vi "GetDeviceReference.vi"(8 "error in (no error)":errorcluster, 10 "Timeout(10s)":i32=10) -> (0 "error out":errorcluster, 3 "MainDevice Reference":refnum<k24>)   [LabVIEW 2019, in "LabNation Scope Driver.lvlib"]
doc: "Acquires the main device reference from the device manager. The reference Identifies the scope for all further actions."
uses:
  LabNation Scope Driver.lvlib
  <vilib>/Utility/error.llb/Error Cluster From Error Code.vi
  <vilib>/ErrorRing/Error Ring.xnode
  C:/Program Files (x86)/LabNation/SmartScope/DeviceInterface.dll
  Program Files (x86)/LabNation/SmartScope/DeviceInterface.dll
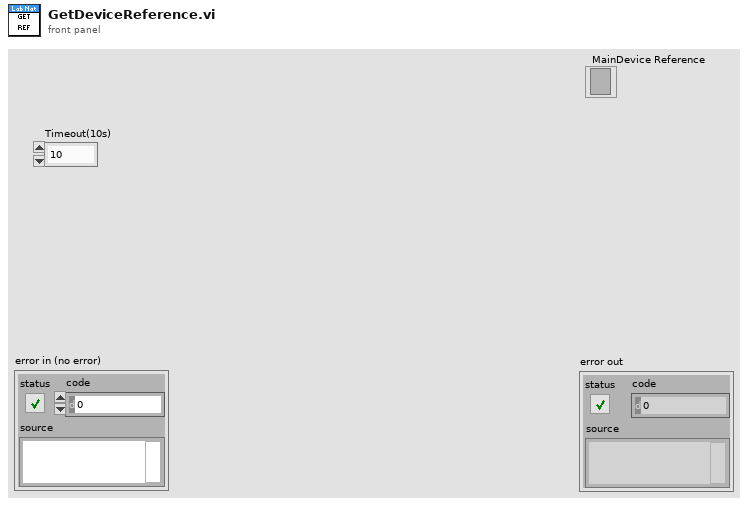
[diagram p1: front panel]
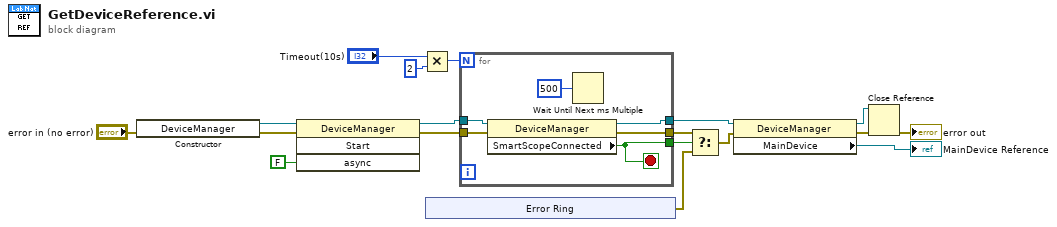
[diagram p0: block diagram]
diagram:
  n1 = constructor class="DeviceManager"(error in="error in (no error)") -> (reference out=w15:refnum<k24>, error out=w14:errorcluster)  [unwired: 2 in, 1 out]
  n2 = invoke class="DeviceManager" method="Start"(reference=w15, error in=w14, "async"=FALSE) -> (reference out=w16:refnum<k24>, error out=w13:errorcluster)  [unwired: 1 in, 2 out]
  n3 = Multiply(x="Timeout(10s)", y=2) -> (x*y=w10:i32)
  n4 = xnode "Error Ring"() -> ("error out"=w1:errorcluster)
  n5 = for {
    N: w10 -> [_]
    tunnel: w16 -> [w24]
    tunnel: [w23] -> w18
    tunnel: w13 -> [w22]
    tunnel: [w21] -> w3
    tunnel: [w19] -> w2
    stop <- w19 stop-if-true
    n6 = property class="DeviceManager"(reference=w24, error in=w22) -> (reference out=w23:refnum<k24>, error out=w21:errorcluster, "SmartScopeConnected"=w19:bool)
    n7 = Wait Until Next ms Multiple(millisecond multiple=u32 500) -> ()  [unwired: 1 out]
  }
  n8 = Select(t=w3, s=w2, f=w1) -> (s? t:f=w4:errorcluster)
  n9 = property class="DeviceManager"(reference=w18, error in=w4) -> (reference out=w6:refnum<k24>, error out=w8:errorcluster, "MainDevice"=→"MainDevice Reference":refnum<k24>)
  n10 = Close Reference(reference=w6, error in (no error)=w8) -> (error out=→"error out":errorcluster)
